vi "בדיקת זמן ניתוק הממסר Mod.vi"(7 "resultUserPrompt":bool, 8 "error":errorcluster, 9 "זמן ניתוק מקסימלי":dbl=0.01 format="%#_13g", 10 "שם הממסר":string="0410-24534 15A ממסר", 11 "Path for Log":path) -> (0 "error out":errorcluster, 1 "בטוח כן/לא":bool, 2 "בדיקת זמן ניתוק הממסר":dbl)   [LabVIEW 2015]
uses:
  <instrlib>/niDMM/nidmm.llb/niDMM Function.ctl
  <instrlib>/niDMM/nidmm.llb/niDMM Resolution in Digits.ctl
  <vilib>/DAQmx/write.llb/DAQmx Write (Digital Bool 1Line 1Point).vi
  <vilib>/DAQmx/create/channels.llb/DAQmx Create Channel (DO-Digital Output).vi
  <vilib>/DAQmx/miscellaneous.llb/DAQmx Fill In Error Info.vi
  <instrlib>/niDMM/nidmm.llb/niDMM Configure Measurement Digits.vi
panel:
  in  "התחל":bool
  # "Right-Click to\nexplain error"
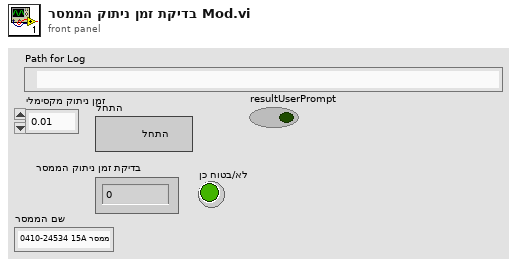
[diagram p1: front panel]
types:
  T1 = enum32{"Invalid", "Standard", "Closed", "Hidden", "Minimized", "Maximized"}
  T2 = typedef "niDMM Function.ctl" = enum16{"DC Volts", "AC Volts", "DC Current", "AC Current", "2-wire Resistance", "4-wire Resistance", "Diode", "Frequency", "Period", "AC Volts DC Coupled", "Capacitance", "Inductance", "Temperature"}
  T3 = typedef "niDMM Resolution in Digits.ctl" = dbl
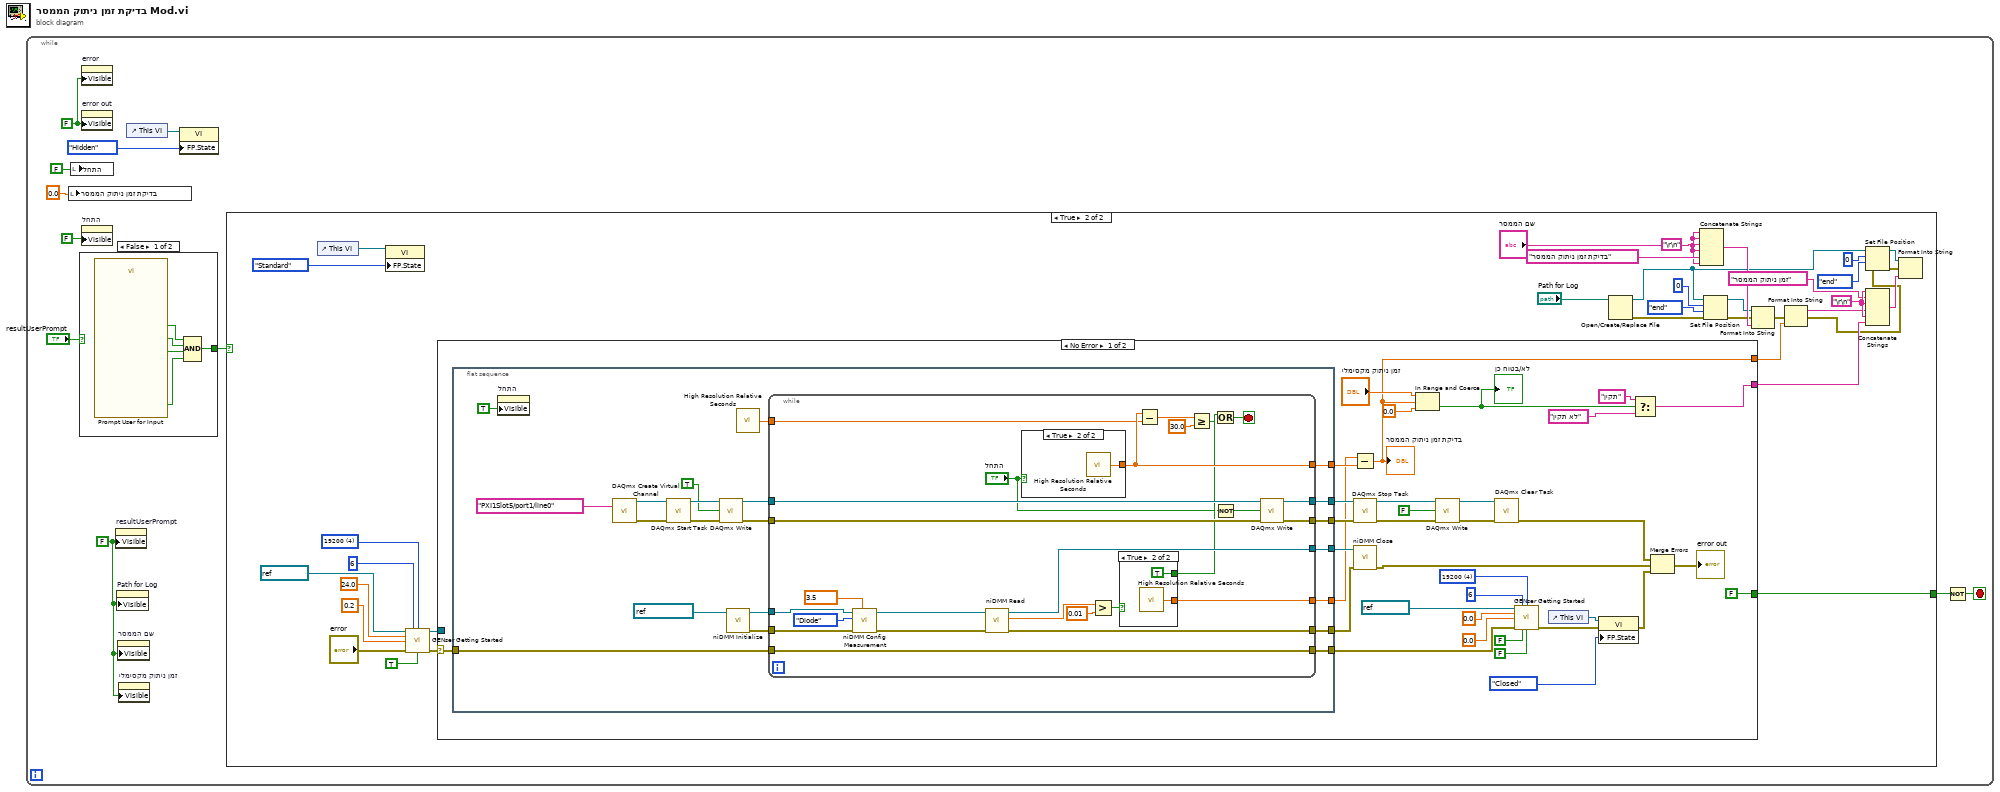
[diagram p0: block diagram]
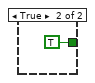
[diagram p2: hidden frame]
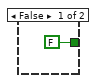
[diagram p3: hidden frame]
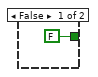
[diagram p4: hidden frame]
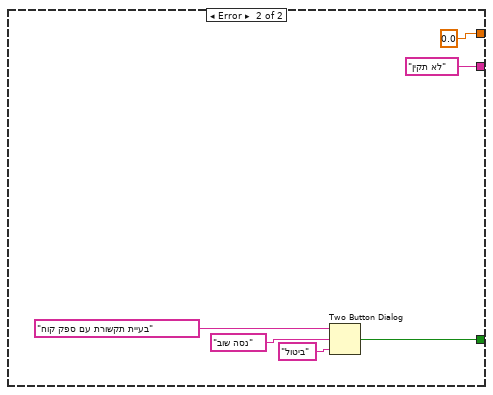
[diagram p6: hidden frame]
diagram:
  n1 = while {
    stop <- w10 stop-if-true
    w1 = FALSE ("Visible")
    w8 = FALSE ("Visible")
    n2 = local write "בדיקת זמן ניתוק הממסר"(0.0 ("זמן ניתוק הממסר")) -> ()
    n3 = local write "התחל"(FALSE ("זמן ניתוק הממסר בטווח כן /לא")) -> ()
    n4 = case shown="False" "resultUserPrompt" {
      tunnel: [w16 TRUE] -> w11
      frame False {
        n5 = call "Prompt User for Input"() -> ("הדקי הרב מודד"=w12:bool, "מגע שלילי"=w13:bool, "מגע חיובי"=w14:bool, "OK"=w15:bool)  [unwired: 15 in, 1 out]
        n6 = Compound Arithmetic op=AND(w15, w14, w13, w12) -> (w16:bool)
      }
      frame True {
      }
    }
    n7 = property on="error" class="Clust (strict)"("Visible"=w8) -> ()  [unwired: 2 in, 2 out]
    n8 = property on="error out" class="Clust (strict)"("Visible"=w8) -> ()  [unwired: 2 in, 2 out]
    n9 = property on="התחל" class="Bool (strict)"("Visible"=FALSE) -> ()  [unwired: 2 in, 2 out]
    n10 = property on="resultUserPrompt" class="Bool (strict)"("Visible"=w1) -> ()  [unwired: 2 in, 2 out]
    n11 = property on="Path for Log" class="Path"("Visible"=w1) -> ()  [unwired: 2 in, 2 out]
    n12 = property on="שם הממסר" class="Str"("Visible"=w1) -> ()  [unwired: 2 in, 2 out]
    n13 = property on="זמן ניתוק מקסימלי" class="DigNum (strict)"("Visible"=w1) -> ()  [unwired: 2 in, 2 out]
    n14 = control-ref of="This VI"() -> (w7:refnum<vi>)
    n15 = property class="VI"(reference=w7, "FP.State"=T1."Hidden" ("Front Panel Window:State")) -> ()  [unwired: 1 in, 2 out]
    n16 = case shown="True" w11 {
      tunnel: [FALSE ("T button?") w46] -> w9
      frame False {
      }
      frame True {
        w27 = "\r\n"
        w35 = "\r\n"
        w50 = u16 4 items=["1200", "2400", "4800", "9600", "19200"] ("BAUD")
        n17 = control-ref of="This VI"() -> (w45:refnum<vi>)
        n18 = property class="VI"(reference=w45, "FP.State"=T1."Standard" ("Front Panel Window:State")) -> ()  [unwired: 1 in, 2 out]
        n19 = call "GENser Getting Started.vi"("VISA"=refnum<visa-resource-name> "COM6", "GEN Addr"=i16 6, "BAUD"=w50, "Voltage Limit"=24.0, "Current Limit"=0.2, "error"="error", "Output On (T)"=TRUE) -> ("VISA out"=w51:refnum<visa-resource-name>, "error out"=w42:errorcluster)  [unwired: 5 in, 2 out]
        n20 = case shown="No Error" w42 {
          selector: w42 -> [w80 _]
          tunnel: w51 -> [_ _]
          tunnel: [FALSE ("T button?") w142] -> w46
          tunnel: [w58 0.0] -> w21
          tunnel: [w54 "לא תקין"] -> w20
          frame No Error {
            w75 = u16 4 items=["1200", "2400", "4800", "9600", "19200"] ("BAUD")
            n21 = flat-sequence {
              tunnel: [w103] -> w59
              tunnel: [w102] -> w60
              tunnel: [w101] -> w67
              tunnel: [w100] -> w68
              tunnel: [w99] -> w64
              tunnel: w80 -> [w97]
              tunnel: [w96] -> w79
              tunnel: [w95] -> w65
              frame #0 {
                n22 = property on="התחל" class="Bool (strict)"("Visible"=TRUE) -> ()  [unwired: 2 in, 2 out]
                n23 = call-poly <vilib>:"DAQmx Create Virtual Channel.vi"("lines"=tag "PXI1Slot5/port1/line0") -> ("task out"=w105:refnum<k21>, "error out"=w106:errorcluster)  [unwired: 13 in]
                n24 = call <vilib>:"DAQmx Start Task.vi"("task/channels in"=w105, "error in"=w106) -> ("task out"=w94:refnum<k21>, "error out"=w93:errorcluster)  [unwired: 12 in]
                n25 = call-poly <vilib>:"DAQmx Write.vi"("task/channels in"=w94, "data"=TRUE, "error in"=w93) -> ("task out"=w91:refnum<k21>, "error out"=w92:errorcluster)  [unwired: 10 in, 1 out]
                n26 = call <instrlib>:"niDMM Initialize.vi"("Instrument Descriptor"=refnum<k15> "PXI1Slot9") -> ("error out"=w107:errorcluster, "instrument handle out"=w108:refnum<k15>)  [unwired: 9 in]
                n27 = call <vilib>:"High Resolution Relative Seconds.vi"() -> ("relative seconds"=w98:dbl)
                n28 = while {
                  tunnel: [w120] -> w102
                  tunnel: [w133] -> w103
                  tunnel: [w122] -> w99
                  tunnel: [w132] -> w100
                  tunnel: [w131] -> w101
                  tunnel: [w121] -> w95
                  tunnel: w108 -> [w126]
                  tunnel: w107 -> [w125]
                  tunnel: w91 -> [w130]
                  tunnel: w92 -> [w129]
                  tunnel: w98 -> [w119]
                  tunnel: [w112] -> w96
                  tunnel: w97 -> [w112]
                  stop <- w116 stop-if-true
                  w135 = T3 3.5 items=["3 1/2"=3.5, "4 1/2"=4.5, "5 1/2"=5.5, "6 1/2"=6.5, "7 1/2"=7.5] ("Resolution in Digits")
                  n29 = call-poly <instrlib>:"niDMM Config Measurement.vi"("Resolution in Digits"=w135, "error in (no error)"=w125, "Function"=niDMM_Function."Diode", "instrument handle"=w126) -> ("error out"=w123:errorcluster, "instrument handle out"=w124:refnum<k15>)  [unwired: 6 in]
                  n30 = call <instrlib>:"niDMM Read.vi"("error in (no error)"=w123, "instrument handle"=w124) -> ("error out"=w121:errorcluster, "Measurement"=w128:dbl, "instrument handle out"=w122:refnum<k15>)  [unwired: 7 in]
                  n31 = case shown="True" "התחל" {
                    tunnel: [_ w139] -> w120
                    frame False {
                    }
                    frame True {
                      n32 = call <vilib>:"High Resolution Relative Seconds.vi"() -> ("relative seconds"=w139:dbl)
                    }
                  }
                  n33 = Greater?(x=w128, y=0.01) -> (0:w113:bool)
                  n34 = case shown="True" w113 {
                    tunnel: [_ w138] -> w133
                    tunnel: [FALSE TRUE] -> w115
                    frame False {
                    }
                    frame True {
                      n35 = call <vilib>:"High Resolution Relative Seconds.vi"() -> ("relative seconds"=w138:dbl)
                    }
                  }
                  n36 = Subtract(x=w120, y=w119) -> (x-y=w118:dbl)
                  n37 = Greater Or Equal?(x=w118, y=30.0) -> (x >= y?=w114:bool)
                  n38 = Or(x=w115, y=w114) -> (x .or. y?=w116:bool)
                  n39 = Not(x="התחל") -> (.not. x?=w111:bool)
                  n40 = call-poly <vilib>:"DAQmx Write.vi"("task/channels in"=w130, "data"=w111, "error in"=w129) -> ("task out"=w132:refnum<k21>, "error out"=w131:errorcluster)  [unwired: 10 in, 1 out]
                }
              }
            }
            n41 = Subtract(x=w59, y=w60) -> (x-y=w58:dbl)
            "בדיקת זמן ניתוק הממסר" <- w58
            n42 = call <vilib>:"DAQmx Stop Task.vi"("task/channels in"=w68, "error in"=w67) -> ("task out"=w73:refnum<k21>, "error out"=w72:errorcluster)  [unwired: 12 in]
            n43 = call <instrlib>:"niDMM Close.vi"("error in (no error)"=w65, "instrument handle"=w64) -> ("error out"=w63:errorcluster)  [unwired: 9 in]
            n44 = In Range and Coerce(upper limit="זמן ניתוק מקסימלי", x=w58, lower limit=0.0) -> (In Range?=w55:bool)  [unwired: 1 out]
            "בטוח כן/לא" <- w55
            n45 = call-poly <vilib>:"DAQmx Write.vi"("task/channels in"=w73, "data"=FALSE, "error in"=w72) -> ("task out"=w70:refnum<k21>, "error out"=w71:errorcluster)  [unwired: 10 in, 1 out]
            n46 = call <vilib>:"DAQmx Clear Task.vi"("task in"=w70, "error in"=w71) -> ("error out"=w66:errorcluster)  [unwired: 13 in]
            n47 = call "GENser Getting Started.vi"("VISA"=refnum<visa-resource-name> "COM6", "GEN Addr"=i16 6, "BAUD"=w75, "Voltage Limit"=0.0, "Current Limit"=0.0, "error"=w79, "Reset (T)"=FALSE ("Output On (T)"), "Output On (T)"=FALSE) -> ("error out"=w81:errorcluster)  [unwired: 4 in, 3 out]
            n48 = control-ref of="This VI"() -> (w83:refnum<vi>)
            n49 = property class="VI"(reference=w83, error in=w81, "FP.State"=T1."Closed" ("Front Panel Window:State")) -> (error out=w77:errorcluster)  [unwired: 1 out]
            n50 = Select(t="תקין", s=w55, f="לא תקין") -> (s? t:f=w54:string)
            n51 = Merge Errors(w66, w63, w77) -> (→"error out":errorcluster)
          }
          frame Error {
            n52 = Two Button Dialog(message="בעיית תקשורת עם ספק קוח", 1:"ביטול" ("F button name (\"Cancel\")"), 2:"נסה שוב" ("T button name (\"OK\")")) -> (T button?=w142:bool)
          }
        }
        n53 = Open/Create/Replace File(file path (use dialog)="Path for Log") -> (refnum out=w22:refnum<file>, error out=w23:errorcluster)  [unwired: 5 in, 1 out]
        n54 = Concatenate Strings(w35, w35, "שם הממסר", w35, "בדיקת זמן ניתוק הממסר", w35) -> (w39:string)
        n55 = Set File Position(offset (in bytes) (0)=i64 0, refnum=w22, from (0:start)=enum16{"start", "end", "current"}."end", error in=w23) -> (refnum out=w36:refnum<file>, error out=w34:errorcluster)
        n56 = Format Into String(initial string=w36, error in=w34, w39) -> (error out=w33:errorcluster)  [unwired: 1 in, 1 out]
        n57 = Format Into String(error in=w33, w21) -> (resulting string=w25:string, error out=w19:errorcluster)  [unwired: 2 in]
        n58 = Set File Position(offset (in bytes) (0)=i64 0, refnum=w22, from (0:start)=enum16{"start", "end", "current"}."end", error in=w19) -> (refnum out=w30:refnum<file>, error out=w31:errorcluster)
        n59 = Concatenate Strings(w27, "זמן ניתוק הממסר", w27, w25, w27, w20) -> (w32:string)
        n60 = Format Into String(initial string=w30, error in=w31, w32) -> ()  [unwired: 1 in, 2 out]
      }
    }
    n61 = Not(x=w9) -> (.not. x?=w10:bool)
  }
